vi "Hybrid Inverter.vi"() -> ()   [LabVIEW 2021]
uses:
  <vilib>/Instr/_visa.llb/VISA Configure Serial Port (Instr).vi
panel:
  out "F-format string":string
  out "KD_TOSET":dbl
  out "KI_TOSET":dbl
  out "KP_TOSET":dbl
  out "closeAPP":bool
  out "CnvrtMode_BOOL":bool
  out "Convrt_Mode_Nr":dbl
  out "COM_ERROR":errorcluster
  out "Pict Ring 10":u16(ring)
  in  "Tab Control":enum32{"Main"}(tab)
  out "KP_CH":dbl format="%.2g"
  out "Ki_CH":dbl format="%.2g"
  out "KD_CH":dbl format="%.2g"
  in  "SET PARAM":bool
  in  "KP SET":dbl
  in  "Ki SET":dbl
  in  "Kd SET":dbl
  out "MCU_AWAKE:":bool
  out "Charging State:":bool
  out "Main Contactor State":bool
  in  "EN_Main_relay":bool
  in  "Set Buck Voltage 3":dbl
  in  "SET_OP_MODE":bool
  in  "Operation Mode":string(combo)
  in  "EMRGNC":bool
  out "Currently Set":dbl
  in  "Tr_RQST":bool
  out "Convrtr_Mode":string
  out "Converter Performance":dbl
  out "Inverter Bus Current":dbl
  out "Battery Bus Current":dbl format="%.2g"
  out "Inverter Bus Voltage":dbl
  out "Battery Bus Voltage":dbl
  out "Pict Ring 9":u16(ring)
  out "Pict Ring 3":u16(ring)
  out "Pict Ring 4":u16(ring)
  out "Pict Ring":u16(ring)
  out "Pict Ring 2":u16(ring)
  out "Pict Ring 11":u16(ring)
  out "Pict Ring 5":u16(ring)
  out "Pict Ring 6":u16(ring)
  out "Pict Ring 7":u16(ring)
  out "Pict Ring 8":u16(ring)
  out "Pict Ring 12":u16(ring)
  in  "Finish":bool
  out "STR_BUF":string
  in  "Start_COM":bool
  in  "VISA_COM":refnum<visa-resource-name>
  in  "Set Buck Voltage":dbl
  in  "Set Buck Voltage 2":dbl
  out "KP_BUCK":dbl format="%.2g"
  out "Ki_BUCK":dbl format="%.2g"
  out "Kd_BUCK":dbl format="%.2g"
  out "Kp BOOST":dbl format="%.2g"
  out "KI BOOST":dbl format="%.2g"
  out "KD BOOST":dbl format="%.2g"
  out "match substring":string
  out "Converter OutPut":dbl
  out "STR_BUF 2":string
  # "Converter Mode:"
  # "Operation Mode:"
  # "Kp"
  # "Ki"
  # "Kd"
  # "Param Config:"
  # "Kp"
  # "Ki"
  # "Kd"
  # "Charger Param:"
  # "Min Battery Voltage:"
  # "Currently Set:"
  # "Converter Performance:"
  # "Inverter Bus Current:"
  # "Battery Bus Current:"
  # "Inverter Bus Voltage:"
  # "Battery Bus Voltage:"
  # "Set Voltage:"
  # "Max Battery Voltage:"
  # "Kp"
  # "Ki"
  # "Kd"
  # "Buck Param:"
  # "Kp"
  # "Ki"
  # "Kd"
  # "Booster Param:"
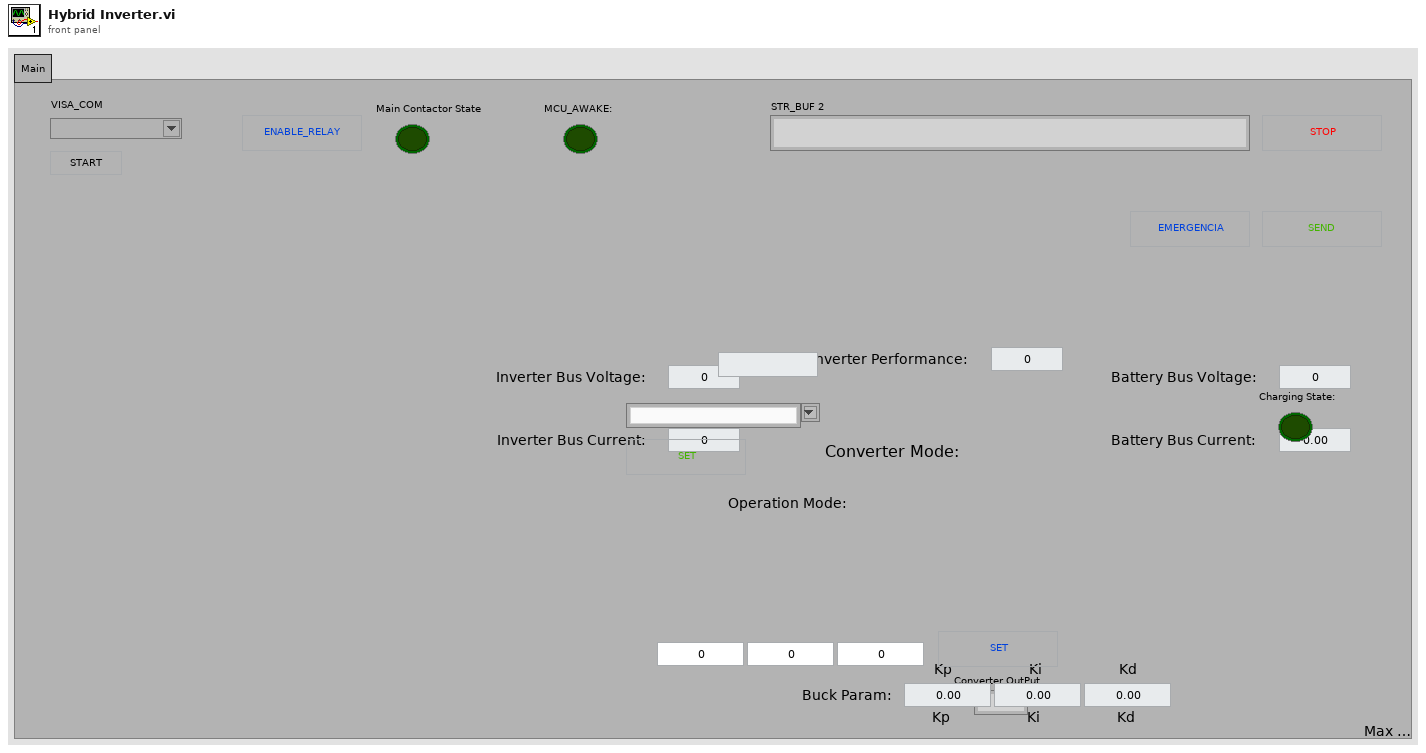
[diagram p1: front panel]
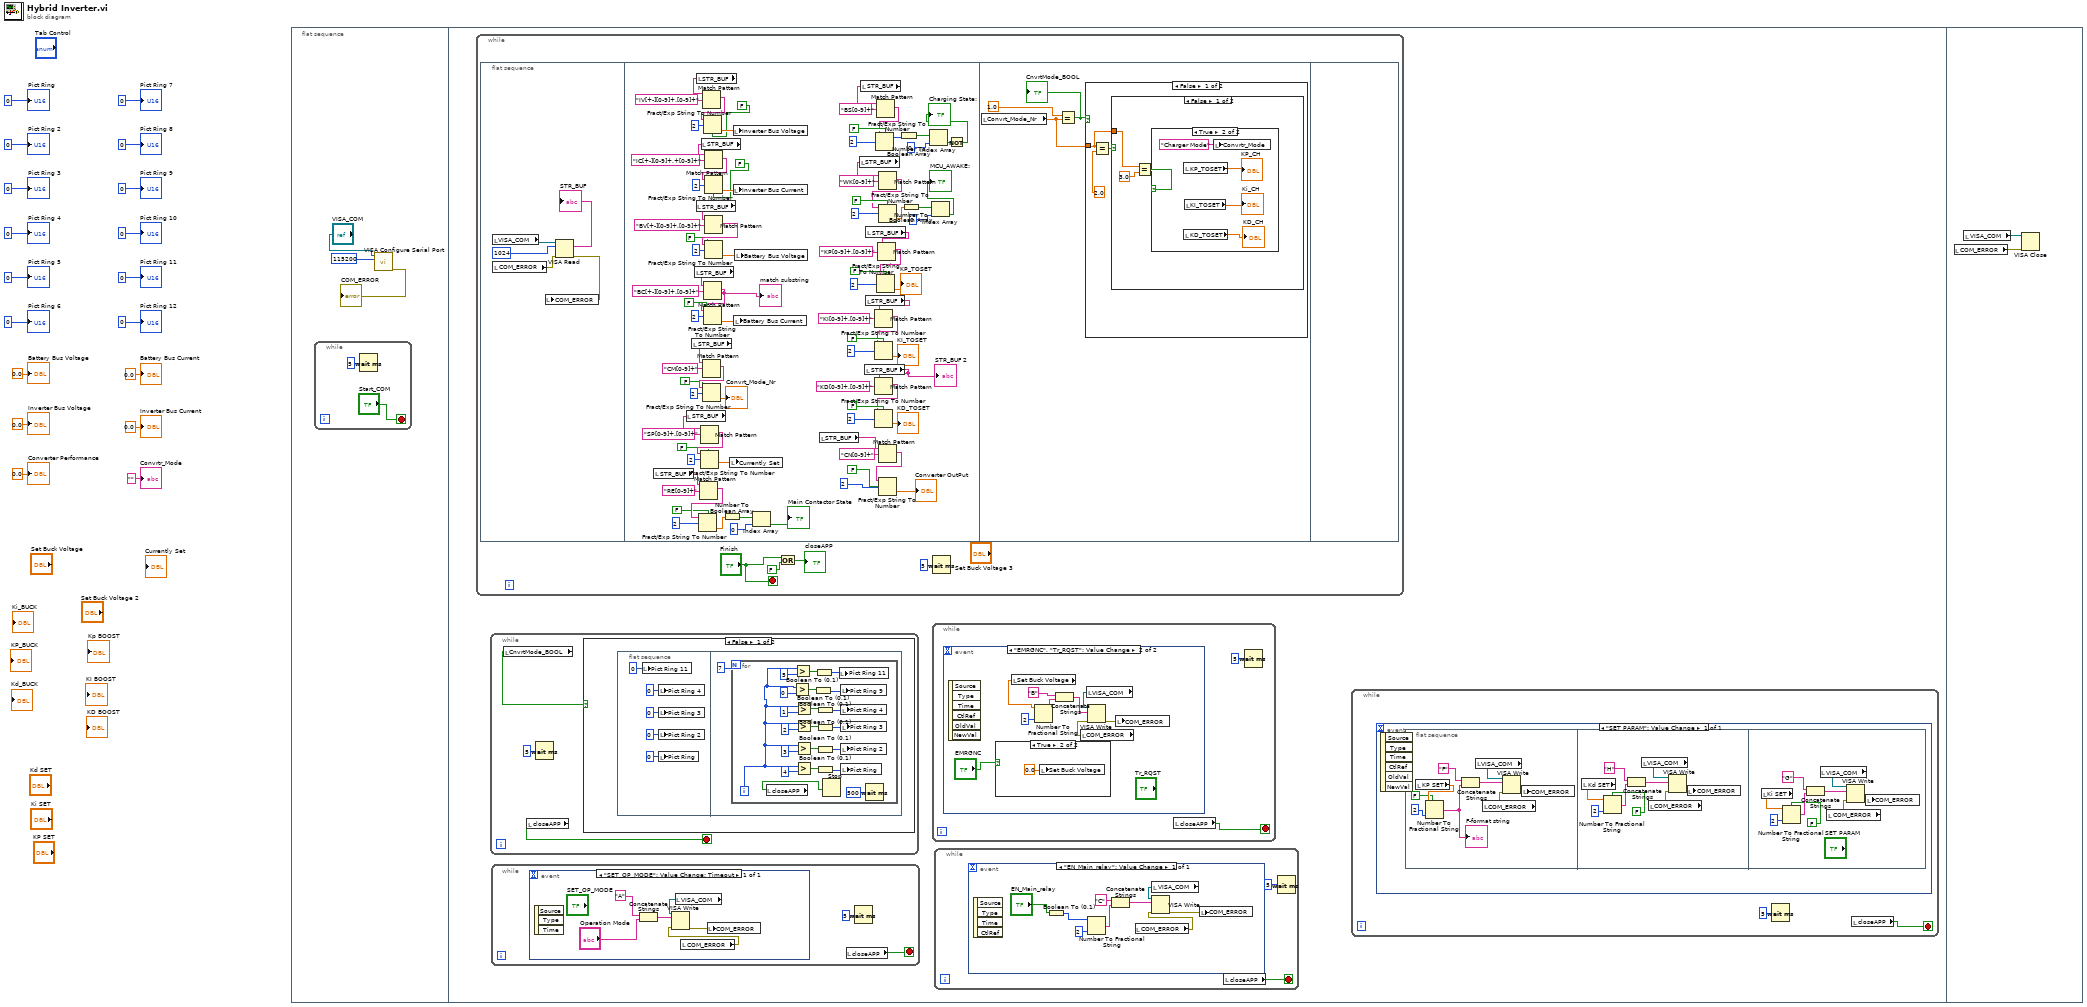
[diagram p0: block diagram]
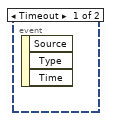
[diagram p2: hidden frame]
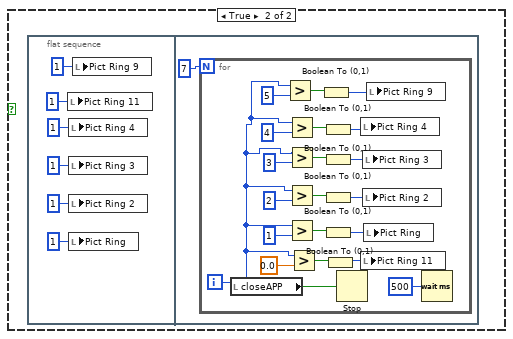
[diagram p4: hidden frame]
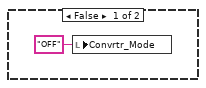
[diagram p5: hidden frame]
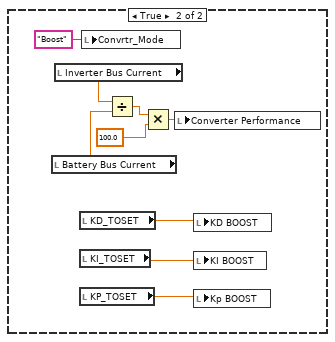
[diagram p6: hidden frame]
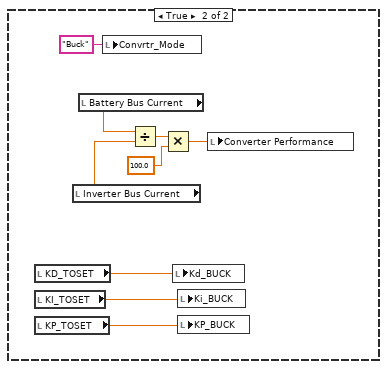
[diagram p7: hidden frame]
diagram:
  n1 = flat-sequence {
    frame #0 {
      n2 = while {
        stop <- "Start_COM" stop-if-true
        n3 = Wait (ms)(milliseconds to wait=u32 5) -> ()  [unwired: 1 out]
      }
      n4 = call-poly "VISA Configure Serial Port"("VISA resource name"="VISA_COM", "baud rate (9600)"=u32 115200) -> ("error out"=→"COM_ERROR":errorcluster)  [unwired: 12 in, 1 out]
    }
    frame #1 {
      n5 = while {
        stop <- "Finish" stop-if-true
        n6 = flat-sequence {
          frame #0 {
            n7 = local read "VISA_COM"() -> (w150:refnum<visa-resource-name>)
            n8 = local read "COM_ERROR"() -> (w148:errorcluster)
            n9 = VISA Read(VISA resource name=w150, byte count=u32 1024, error in (no error)=w148) -> (read buffer=→"STR_BUF":string, error out=w146:errorcluster)  [unwired: 2 out]
            n10 = local write "COM_ERROR"(w146) -> ()
          }
          frame #1 {
            n11 = local read "STR_BUF"() -> (w195:string)
            n12 = local read "STR_BUF"() -> (w208:string)
            n13 = local read "STR_BUF"() -> (w216:string)
            n14 = local read "STR_BUF"() -> (w215:string)
            n15 = local read "STR_BUF"() -> (w214:string)
            n16 = local read "STR_BUF"() -> (w237:string)
            n17 = Match Pattern(string=w195, regular expression="RE[0-9]+") -> (match substring=w202:string)  [unwired: 1 in, 3 out]
            n18 = Fract/Exp String To Number(use system decimal point (T)=FALSE, string=w202, offset=2) -> (number=w194:dbl)  [unwired: 1 in, 1 out]
            n19 = Match Pattern(string=w208, regular expression="SP[0-9]+.[0-9]+") -> (match substring=w206:string)  [unwired: 1 in, 3 out]
            n20 = Fract/Exp String To Number(use system decimal point (T)=FALSE, string=w206, offset=2) -> (number=w203:dbl)  [unwired: 1 in, 1 out]
            n21 = local read "STR_BUF"() -> (w217:string)
            n22 = Match Pattern(string=w216, regular expression="CM[0-9]+") -> (match substring=w222:string)  [unwired: 1 in, 3 out]
            n23 = Fract/Exp String To Number(use system decimal point (T)=FALSE, string=w222, offset=2) -> (number=→"Convrt_Mode_Nr":dbl)  [unwired: 1 in, 1 out]
            n24 = Match Pattern(string=w237, regular expression="IV[+-][0-9]+.[0-9]+") -> (match substring=w235:string)  [unwired: 1 in, 3 out]
            n25 = Fract/Exp String To Number(use system decimal point (T)=FALSE, string=w235, offset=2) -> (number=w233:dbl)  [unwired: 1 in, 1 out]
            n26 = Match Pattern(string=w215, regular expression="BC[+-][0-9]+.[0-9]+") -> (match substring=w158:string)  [unwired: 1 in, 3 out]
            "match substring" <- w158
            n27 = Fract/Exp String To Number(use system decimal point (T)=FALSE, string=w158, offset=2) -> (number=w224:dbl)  [unwired: 1 in, 1 out]
            n28 = Match Pattern(string=w217, regular expression="IC[+-][0-9]+.+[0-9]+") -> (match substring=w232:string)  [unwired: 1 in, 3 out]
            n29 = Fract/Exp String To Number(use system decimal point (T)=FALSE, string=w232, offset=2) -> (number=w223:dbl)  [unwired: 1 in, 1 out]
            n30 = Match Pattern(string=w214, regular expression="BV[+-][0-9]+.[0-9]+") -> (match substring=w230:string)  [unwired: 1 in, 3 out]
            n31 = Fract/Exp String To Number(use system decimal point (T)=FALSE, string=w230, offset=2) -> (number=w225:dbl)  [unwired: 1 in, 1 out]
            n32 = Number To Boolean Array(number=w194) -> (Boolean array=w198:bool[])
            n33 = local write "Currently Set"(w203) -> ()
            n34 = local write "Inverter Bus Voltage"(w233) -> ()
            n35 = local write "Inverter Bus Current"(w223) -> ()
            n36 = local write "Battery Bus Current"(w224) -> ()
            n37 = local write "Battery Bus Voltage"(w225) -> ()
            n38 = Index Array(array=w198, index=0) -> (element=→"Main Contactor State":bool)
            n39 = local read "STR_BUF"() -> (w151:string)
            n40 = local read "STR_BUF"() -> (w182:string)
            n41 = local read "STR_BUF"() -> (w187:string)
            n42 = local read "STR_BUF"() -> (w153:string)
            "STR_BUF 2" <- w153
            n43 = local read "STR_BUF"() -> (w166:string)
            n44 = local read "STR_BUF"() -> (w165:string)
            n45 = Match Pattern(string=w166, regular expression="KI[0-9]+.[0-9]+") -> (match substring=w163:string)  [unwired: 1 in, 3 out]
            n46 = Fract/Exp String To Number(use system decimal point (T)=FALSE, string=w163, offset=2) -> (number=→"KI_TOSET":dbl)  [unwired: 1 in, 1 out]
            n47 = Match Pattern(string=w153, regular expression="KD[0-9]+.[0-9]+") -> (match substring=w162:string)  [unwired: 1 in, 3 out]
            n48 = Fract/Exp String To Number(use system decimal point (T)=FALSE, string=w162, offset=2) -> (number=→"KD_TOSET":dbl)  [unwired: 1 in, 1 out]
            n49 = Match Pattern(string=w187, regular expression="BS[0-9]+") -> (match substring=w191:string)  [unwired: 1 in, 3 out]
            n50 = Fract/Exp String To Number(use system decimal point (T)=FALSE, string=w191, offset=2) -> (offset past number=w190:i32)  [unwired: 1 in, 1 out]
            n51 = Match Pattern(string=w165, regular expression="KP[0-9]+.[0-9]+") -> (match substring=w164:string)  [unwired: 1 in, 3 out]
            n52 = Fract/Exp String To Number(use system decimal point (T)=FALSE, string=w164, offset=2) -> (number=→"KP_TOSET":dbl)  [unwired: 1 in, 1 out]
            n53 = Match Pattern(string=w182, regular expression="WK[0-9]+") -> (match substring=w181:string)  [unwired: 1 in, 3 out]
            n54 = Fract/Exp String To Number(use system decimal point (T)=FALSE, string=w181, offset=2) -> (number=w176:dbl)  [unwired: 1 in, 1 out]
            n55 = Match Pattern(string=w151, regular expression="CN[0-9]+") -> (match substring=w157:string)  [unwired: 1 in, 3 out]
            n56 = Fract/Exp String To Number(use system decimal point (T)=FALSE, string=w157, offset=2) -> (number=→"Converter OutPut":dbl)  [unwired: 1 in, 1 out]
            n57 = Number To Boolean Array(number=w190) -> (Boolean array=w189:bool[])
            n58 = Number To Boolean Array(number=w176) -> (Boolean array=w180:bool[])
            n59 = Index Array(array=w189, index=0) -> (element=w185:bool)
            "Charging State:" <- w185
            n60 = Index Array(array=w180, index=0) -> (element=→"MCU_AWAKE:":bool)
            n61 = Not(x=w185) -> ()  [unwired: 1 out]
          }
          frame #2 {
            n62 = local read "Convrt_Mode_Nr"() -> (w238:dbl)
            n63 = Equal?(x=1.0, y=w238) -> (x = y?=w240:bool)
            "CnvrtMode_BOOL" <- w240
            n64 = case shown="False" w240 {
              tunnel: w238 -> [w241 _]
              frame False {
                n65 = Equal?(x=w241, y=2.0) -> (x = y?=w243:bool)
                n66 = case shown="False" w243 {
                  tunnel: w241 -> [w246 _]
                  frame False {
                    n67 = Equal?(x=w246, y=3.0) -> (x = y?=w244:bool)
                    n68 = case shown="True" w244 {
                      frame False {
                        n69 = local write "Convrtr_Mode"("OFF" ("Convrtr_Mode")) -> ()
                      }
                      frame True {
                        n70 = local read "KP_TOSET"() -> (→"KP_CH":dbl)
                        n71 = local read "KD_TOSET"() -> (→"KD_CH":dbl)
                        n72 = local read "KI_TOSET"() -> (→"Ki_CH":dbl)
                        n73 = local write "Convrtr_Mode"("Charger Mode" ("Convrtr_Mode")) -> ()
                      }
                    }
                  }
                  frame True {
                    n74 = local read "Battery Bus Current"() -> (w259:dbl)
                    n75 = local read "Inverter Bus Current"() -> (w258:dbl)
                    n76 = local read "KD_TOSET"() -> (w252:dbl)
                    n77 = local read "KI_TOSET"() -> (w253:dbl)
                    n78 = local read "KP_TOSET"() -> (w254:dbl)
                    n79 = local write "Convrtr_Mode"("Boost" ("Convrtr_Mode")) -> ()
                    n80 = Divide(x=w258, y=w259) -> (x/y=w256:dbl)
                    n81 = Multiply(x=w256, y=100.0) -> (x*y=w257:dbl)
                    n82 = local write "Converter Performance"(w257) -> ()
                    n83 = local write "KD BOOST"(w252) -> ()
                    n84 = local write "KI BOOST"(w253) -> ()
                    n85 = local write "Kp BOOST"(w254) -> ()
                  }
                }
              }
              frame True {
                n86 = local read "KD_TOSET"() -> (w263:dbl)
                n87 = local read "KI_TOSET"() -> (w262:dbl)
                n88 = local read "KP_TOSET"() -> (w261:dbl)
                n89 = local read "Inverter Bus Current"() -> (w266:dbl)
                n90 = local read "Battery Bus Current"() -> (w267:dbl)
                n91 = local write "Convrtr_Mode"("Buck" ("Convrtr_Mode")) -> ()
                n92 = Divide(x=w267, y=w266) -> (x/y=w268:dbl)
                n93 = Multiply(x=w268, y=100.0) -> (x*y=w265:dbl)
                n94 = local write "Kd_BUCK"(w263) -> ()
                n95 = local write "Ki_BUCK"(w262) -> ()
                n96 = local write "KP_BUCK"(w261) -> ()
                n97 = local write "Converter Performance"(w265) -> ()
              }
            }
          }
          frame #3 {
          }
        }
        n98 = Or(x="Finish", y=FALSE) -> (x .or. y?=→"closeAPP":bool)
        n99 = Wait (ms)(milliseconds to wait=u32 5) -> ()  [unwired: 1 out]
      }
      n100 = while {
        stop <- w84 stop-if-true
        n101 = local read "CnvrtMode_BOOL"() -> (w86:bool)
        n102 = local read "closeAPP"() -> (w84:bool)
        n103 = Wait (ms)(milliseconds to wait=u32 5) -> ()  [unwired: 1 out]
        n104 = case shown="False" w86 {
          frame False {
            n105 = flat-sequence {
              frame #0 {
                n106 = local write "Pict Ring 11"(u16 0 ("Pict Ring 11")) -> ()
                n107 = local write "Pict Ring 4"(u16 0 ("Pict Ring 4")) -> ()
                n108 = local write "Pict Ring 3"(u16 0 ("Pict Ring 3")) -> ()
                n109 = local write "Pict Ring 2"(u16 0 ("Pict Ring 2")) -> ()
                n110 = local write "Pict Ring"(u16 0 ("Pict Ring")) -> ()
              }
              frame #1 {
                n111 = for {
                  N: 7 -> [_]
                  i -> [w95]
                  n112 = local read "closeAPP"() -> (w97:bool)
                  n113 = Greater?(x=w95, y=0) -> (0:w100:bool)
                  n114 = Greater?(x=w95, y=5) -> (0:w96:bool)
                  n115 = Greater?(x=w95, y=1) -> (0:w113:bool)
                  n116 = Greater?(x=w95, y=2) -> (0:w111:bool)
                  n117 = Greater?(x=w95, y=3) -> (0:w110:bool)
                  n118 = Greater?(x=w95, y=4) -> (0:w109:bool)
                  n119 = Boolean To (0,1)(Boolean=w100) -> (0, 1=w99:i16)
                  n120 = Boolean To (0,1)(Boolean=w96) -> (0, 1=w93:i16)
                  n121 = Boolean To (0,1)(Boolean=w113) -> (0, 1=w112:i16)
                  n122 = Boolean To (0,1)(Boolean=w111) -> (0, 1=w106:i16)
                  n123 = Boolean To (0,1)(Boolean=w110) -> (0, 1=w107:i16)
                  n124 = Boolean To (0,1)(Boolean=w109) -> (0, 1=w108:i16)
                  n125 = Stop(stop? (T)=w97) -> ()
                  n126 = local write "Pict Ring 11"(w93) -> ()
                  n127 = local write "Pict Ring 9"(w99) -> ()
                  n128 = local write "Pict Ring 4"(w112) -> ()
                  n129 = local write "Pict Ring 3"(w106) -> ()
                  n130 = local write "Pict Ring 2"(w107) -> ()
                  n131 = local write "Pict Ring"(w108) -> ()
                  n132 = Wait (ms)(milliseconds to wait=u32 500) -> ()  [unwired: 1 out]
                }
              }
            }
          }
          frame True {
            n133 = flat-sequence {
              frame #0 {
                n134 = local write "Pict Ring 11"(u16 1 ("Pict Ring 11")) -> ()
                n135 = local write "Pict Ring 4"(u16 1 ("Pict Ring 4")) -> ()
                n136 = local write "Pict Ring 3"(u16 1 ("Pict Ring 3")) -> ()
                n137 = local write "Pict Ring 2"(u16 1 ("Pict Ring 2")) -> ()
                n138 = local write "Pict Ring"(u16 1 ("Pict Ring")) -> ()
                n139 = local write "Pict Ring 9"(u16 1 ("Pict Ring 9")) -> ()
              }
              frame #1 {
                n140 = for {
                  N: 7 -> [_]
                  i -> [w122]
                  n141 = local read "closeAPP"() -> (w125:bool)
                  n142 = Greater?(x=w122, y=5) -> (0:w128:bool)
                  n143 = Greater?(x=w122, y=4) -> (0:w141:bool)
                  n144 = Greater?(x=w122, y=3) -> (0:w140:bool)
                  n145 = Greater?(x=w122, y=2) -> (0:w139:bool)
                  n146 = Greater?(x=w122, y=1) -> (0:w138:bool)
                  n147 = Greater?(x=w122, y=0.0) -> (0:w124:bool)
                  n148 = Boolean To (0,1)(Boolean=w128) -> (0, 1=w127:i16)
                  n149 = Boolean To (0,1)(Boolean=w141) -> (0, 1=w133:i16)
                  n150 = Boolean To (0,1)(Boolean=w140) -> (0, 1=w132:i16)
                  n151 = Boolean To (0,1)(Boolean=w139) -> (0, 1=w131:i16)
                  n152 = Boolean To (0,1)(Boolean=w138) -> (0, 1=w130:i16)
                  n153 = Boolean To (0,1)(Boolean=w124) -> (0, 1=w121:i16)
                  n154 = Stop(stop? (T)=w125) -> ()
                  n155 = local write "Pict Ring 4"(w133) -> ()
                  n156 = local write "Pict Ring 11"(w121) -> ()
                  n157 = local write "Pict Ring 3"(w132) -> ()
                  n158 = local write "Pict Ring 2"(w131) -> ()
                  n159 = local write "Pict Ring"(w130) -> ()
                  n160 = local write "Pict Ring 9"(w127) -> ()
                  n161 = Wait (ms)(milliseconds to wait=u32 500) -> ()  [unwired: 1 out]
                }
              }
            }
          }
        }
      }
      n162 = while {
        stop <- w65 stop-if-true
        n163 = event shown="[0] \"SET_OP_MODE\": Value Change;  Timeout" {
          selector: _ -> [_]
          dyn-events: _ -> [_]
          timeout: _ -> [_]
          event "SET_OP_MODE": Value Change; Timeout {
            n164 = event-data() -> ()  [unwired: 1 in, 3 out]
            n165 = Concatenate Strings("A" ("string"), "Operation Mode") -> (w68:string)
            n166 = local read "VISA_COM"() -> (w69:refnum<visa-resource-name>)
            n167 = local read "COM_ERROR"() -> (w71:errorcluster)
            n168 = VISA Write(VISA resource name=w69, write buffer=w68, error in (no error)=w71) -> (error out=w70:errorcluster)  [unwired: 2 out]
            n169 = local write "COM_ERROR"(w70) -> ()
          }
        }
        n170 = local read "closeAPP"() -> (w65:bool)
        n171 = Wait (ms)(milliseconds to wait=u32 5) -> ()  [unwired: 1 out]
      }
      n172 = while {
        stop <- w73 stop-if-true
        n173 = event shown="[1] \"EMRGNC\", \"Tr_RQST\": Value Change" {
          selector: _ -> [_ _]
          dyn-events: _ -> [_ _]
          timeout: _ -> [_ _]
          event Timeout {
            n174 = event-data() -> ()  [unwired: 1 in, 3 out]
          }
          event "EMRGNC", "Tr_RQST": Value Change {
            n175 = event-data() -> ()  [unwired: 1 in, 6 out]
            n176 = case shown="True" "EMRGNC" {
              frame False {
              }
              frame True {
                n177 = local write "Set Buck Voltage"(0.0 ("Set Buck Voltage")) -> ()
              }
            }
            n178 = local read "Set Buck Voltage"() -> (w82:dbl)
            n179 = Number To Fractional String(number=w82, precision (6)=i16 2) -> (F-format string=w76:string)  [unwired: 2 in]
            n180 = Concatenate Strings("B" ("string"), w76) -> (w75:string)
            n181 = local read "COM_ERROR"() -> (w79:errorcluster)
            n182 = local read "VISA_COM"() -> (w80:refnum<visa-resource-name>)
            n183 = VISA Write(VISA resource name=w80, write buffer=w75, error in (no error)=w79) -> (error out=w77:errorcluster)  [unwired: 2 out]
            n184 = local write "COM_ERROR"(w77) -> ()
          }
        }
        n185 = local read "closeAPP"() -> (w73:bool)
        n186 = Wait (ms)(milliseconds to wait=u32 5) -> ()  [unwired: 1 out]
      }
      n187 = while {
        stop <- w53 stop-if-true
        n188 = event shown="[0] \"EN_Main_relay\": Value Change" {
          selector: _ -> [_]
          dyn-events: _ -> [_]
          timeout: _ -> [_]
          event "EN_Main_relay": Value Change {
            n189 = event-data() -> ()  [unwired: 1 in, 4 out]
            n190 = Boolean To (0,1)(Boolean="EN_Main_relay") -> (0, 1=w56:i16)
            n191 = Number To Fractional String(number=w56, precision (6)=i16 2) -> (F-format string=w63:string)  [unwired: 2 in]
            n192 = Concatenate Strings("C" ("string"), w63) -> (w61:string)
            n193 = local read "COM_ERROR"() -> (w60:errorcluster)
            n194 = local read "VISA_COM"() -> (w58:refnum<visa-resource-name>)
            n195 = VISA Write(VISA resource name=w58, write buffer=w61, error in (no error)=w60) -> (error out=w59:errorcluster)  [unwired: 2 out]
            n196 = local write "COM_ERROR"(w59) -> ()
          }
        }
        n197 = local read "closeAPP"() -> (w53:bool)
        n198 = Wait (ms)(milliseconds to wait=u32 5) -> ()  [unwired: 1 out]
      }
      n199 = while {
        stop <- w25 stop-if-true
        n200 = event shown="[0] \"SET PARAM\": Value Change" {
          selector: _ -> [_]
          dyn-events: _ -> [_]
          timeout: _ -> [_]
          event "SET PARAM": Value Change {
            n201 = event-data() -> ()  [unwired: 1 in, 6 out]
            n202 = flat-sequence {
              frame #0 {
                n203 = local read "KP SET"() -> (w27:dbl)
                n204 = Number To Fractional String(use system decimal point (T)=FALSE, number=w27, precision (6)=i16 2) -> (F-format string=w33:string)  [unwired: 1 in]
                "F-format string" <- w33
                n205 = Concatenate Strings("F" ("string"), w33) -> (w32:string)
                n206 = local read "VISA_COM"() -> (w28:refnum<visa-resource-name>)
                n207 = local read "COM_ERROR"() -> (w30:errorcluster)
                n208 = VISA Write(VISA resource name=w28, write buffer=w32, error in (no error)=w30) -> (error out=w31:errorcluster)  [unwired: 2 out]
                n209 = local write "COM_ERROR"(w31) -> ()
              }
              frame #1 {
                n210 = local read "Kd SET"() -> (w42:dbl)
                n211 = Number To Fractional String(use system decimal point (T)=FALSE, number=w42, precision (6)=i16 2) -> (F-format string=w38:string)  [unwired: 1 in]
                n212 = Concatenate Strings("H" ("string"), w38) -> (w39:string)
                n213 = local read "VISA_COM"() -> (w43:refnum<visa-resource-name>)
                n214 = local read "COM_ERROR"() -> (w41:errorcluster)
                n215 = VISA Write(VISA resource name=w43, write buffer=w39, error in (no error)=w41) -> (error out=w40:errorcluster)  [unwired: 2 out]
                n216 = local write "COM_ERROR"(w40) -> ()
              }
              frame #2 {
                n217 = local read "Ki SET"() -> (w51:dbl)
                n218 = Number To Fractional String(use system decimal point (T)=FALSE, number=w51, precision (6)=i16 2) -> (F-format string=w47:string)  [unwired: 1 in]
                n219 = Concatenate Strings("G" ("string"), w47) -> (w48:string)
                n220 = local read "VISA_COM"() -> (w52:refnum<visa-resource-name>)
                n221 = local read "COM_ERROR"() -> (w50:errorcluster)
                n222 = VISA Write(VISA resource name=w52, write buffer=w48, error in (no error)=w50) -> (error out=w49:errorcluster)  [unwired: 2 out]
                n223 = local write "COM_ERROR"(w49) -> ()
              }
            }
          }
        }
        n224 = Wait (ms)(milliseconds to wait=u32 5) -> ()  [unwired: 1 out]
        n225 = local read "closeAPP"() -> (w25:bool)
      }
    }
    frame #2 {
      n226 = local read "COM_ERROR"() -> (w270:errorcluster)
      n227 = local read "VISA_COM"() -> (w271:refnum<visa-resource-name>)
      n228 = VISA Close(VISA resource name=w271, error in (no error)=w270) -> ()  [unwired: 1 out]
    }
  }
  "Pict Ring 9" <- u16 0 ("Pict Ring 9")
  "Pict Ring 10" <- u16 0 ("Pict Ring 10")
  "Pict Ring 11" <- u16 0 ("Pict Ring 11")
  "Pict Ring 5" <- u16 0 ("Pict Ring 5")
  "Pict Ring 6" <- u16 0 ("Pict Ring 6")
  "Pict Ring 7" <- u16 0 ("Pict Ring 7")
  "Pict Ring 8" <- u16 0 ("Pict Ring 8")
  "Pict Ring 12" <- u16 0 ("Pict Ring 12")
  "Battery Bus Voltage" <- 0.0 ("Battery Bus Voltage")
  "Inverter Bus Voltage" <- 0.0 ("Inverter Bus Voltage")
  "Battery Bus Current" <- 0.0 ("Battery Bus Current")
  "Inverter Bus Current" <- 0.0 ("Inverter Bus Current")
  "Converter Performance" <- 0.0 ("Converter Performance")
  "Convrtr_Mode" <- "" ("Convrtr_Mode")
  "Pict Ring" <- u16 0 ("Pict Ring")
  "Pict Ring 2" <- u16 0 ("Pict Ring 2")
  "Pict Ring 3" <- u16 0 ("Pict Ring 3")
  "Pict Ring 4" <- u16 0 ("Pict Ring 4")
